vi "DoubleClick.vi"(4 "Point":cluster{"H":T1, "V":T1}, 5 "XRef":refnum<vi>, 6 "State In":T2) -> (0 "Reply":string[](array[string]), 2 "State Out":T2)   [LabVIEW 2015, in "Async-Or-Show.xnode"]
doc: "This ability VI is called when the user double clicks on your XNode. Point is the the location on the XNode that the user clicked relative to the top-left corner of the XNode. A common pattern is to open a configuration dialog when the user double clicks on an XNode, but you may choose to behave differently. Use Reply to inform LabVIEW of any actions it needs to take.\n\nDefault behavior: None.\n\nThis ability provides UI and OS messages are handled."
uses:
  Async-Or-Show.xnode
  State.ctl
  <vilib>/Utility/miscctls.llb/LVRectTypeDef.ctl
  <vilib>/picture/picture.llb/imagedata.ctl
  <vilib>/XNodeSupport/XNodeInt.ctl
  <vilib>/XNodeSupport/NI_XNodeSupport.lvlib
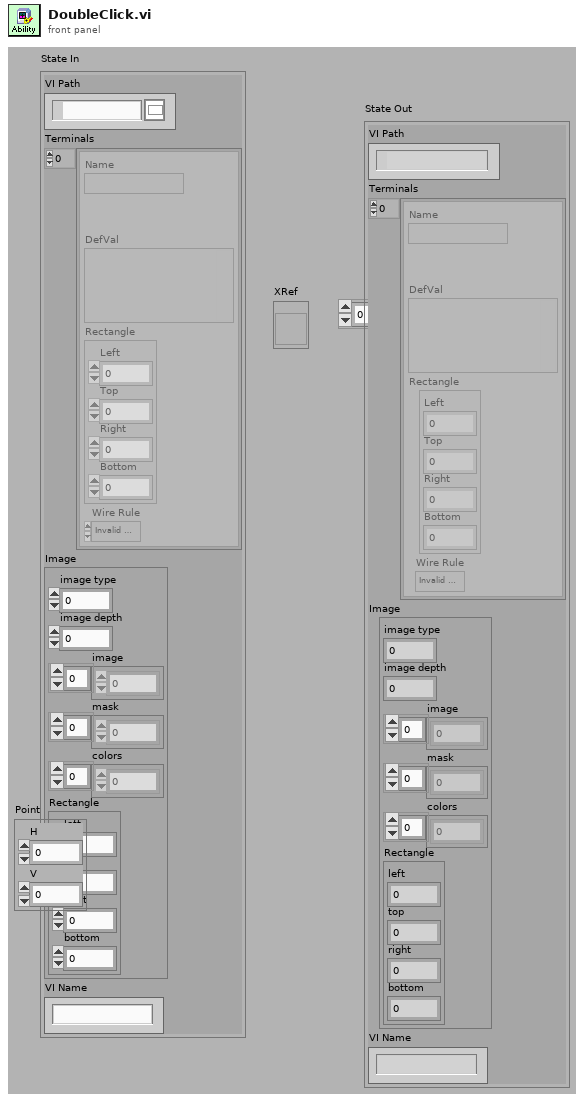
[diagram p1: front panel]
types:
  T1 = typedef "NI_XNodeSupport.lvlib/XNodeInt.ctl" = i32
  T2 = typedef "Async-Or-Show.xnode/State.ctl" = cluster{"VI Path":path, "Terminals":cluster{"Name":string, "DefVal":variant, "Rectangle":T3, "Wire Rule":enum16{"Invalid Wire Rule", "Required", "Recommended", "Optional", "Dynamic Dispatch"}}[], "Image":T4, "VI Name":string}
  T3 = typedef "LVRectTypeDef.ctl" = cluster{"Left":i16, "Top":i16, "Right":i16, "Bottom":i16}
  T4 = typedef "imagedata.ctl" = cluster{"image type":i32, "image depth":i32, "image":u8[], "mask":u8[], "colors":u32[], "Rectangle":cluster{"left":i16, "top":i16, "right":i16, "bottom":i16}}
  T5 = enum16{"Invalid Wire Rule", "Required", "Recommended", "Optional", "Dynamic Dispatch"}[]
  T6 = cluster{"Name":string, "DefVal":variant, "Rectangle":T3, "Wire Rule":enum16{"Invalid Wire Rule", "Required", "Recommended", "Optional", "Dynamic Dispatch"}}[]
  T7 = cluster{"Label.Text":string, "DefVal":variant, "Rectangle":T3, "Wire Rule":enum16{"Invalid Wire Rule", "Required", "Recommended", "Optional", "Dynamic Dispatch"}}[]
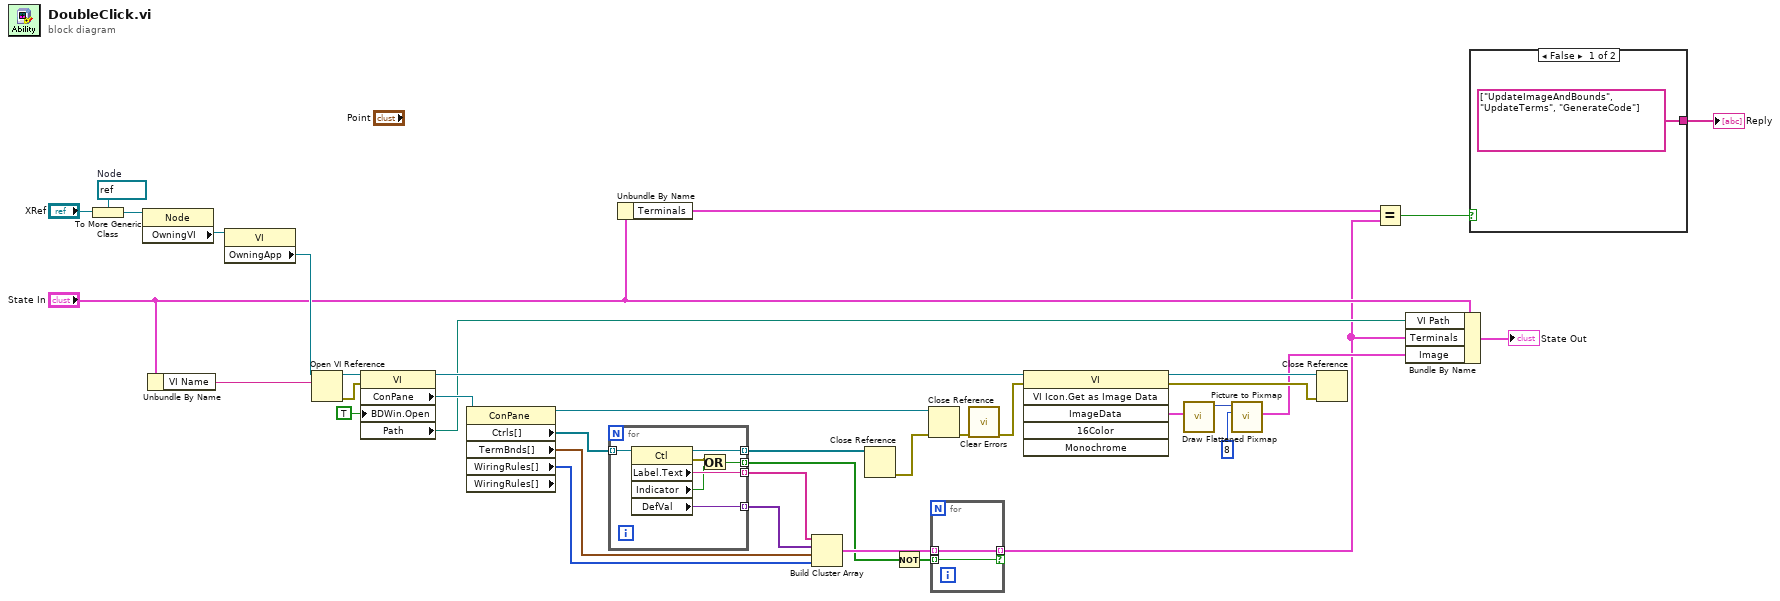
[diagram p0: block diagram]
diagram:
  w31 = refnum<vi> refnum  # Node
  n1 = To More Generic Class(target class=w31, reference="XRef") -> (generic class reference=w30:refnum<vi>)
  n2 = property class="Node"(reference=w30) -> ("OwningVI"=w29:refnum<vi>)  [unwired: 1 in, 2 out]
  n3 = Unbundle By Name("State In") -> ("VI Name"=w34:string)
  n4 = property class="VI"(reference=w29) -> ("OwningApp"=w28:refnum<vi>)  [unwired: 1 in, 2 out]
  n5 = Open VI Reference(application reference (local)=w28, vi path=w34) -> (vi reference=w37:refnum<vi>, error out=w36:errorcluster)  [unwired: 4 in]
  n6 = property class="VI"(reference=w37, error in=w36, "BDWin.Open"=TRUE ("Block Diagram Window:Open")) -> (reference out=w9:refnum<vi>, "ConPane"=w8:refnum<vi>, "Path"=w6:path)  [unwired: 1 out]
  n7 = property class="ConPane" props=["Ctrls[]", "TermBnds[]", "WiringRules[]", "WiringRules[]"](reference=w8) -> (reference out=w16:refnum<vi>, "Ctrls[]"=w27:refnum<vi>[], "TermBnds[]"=w25:T3[], "WiringRules[]"=w26:T5)  [unwired: 1 in, 2 out]
  n8 = for {
    tunnel: w27 -> [w44] mode=indexing
    tunnel: [w43] -> w23 mode=indexing
    tunnel: [w42] -> w24 mode=indexing
    tunnel: [w41] -> w22 mode=indexing
    tunnel: [w38] -> w14 mode=indexing
    n9 = property class="Ctl"(reference=w44) -> (reference out=w41:refnum<vi>, error out=w40:errorcluster, "Label.Text"=w43:string, "Indicator"=w39:bool, "DefVal"=w42:variant)  [unwired: 1 in]
    n10 = Or(x=w40, y=w39) -> (x .or. y?=w38:bool)
  }
  n11 = Unbundle By Name("State In") -> ("Terminals"=w5:T6)
  n12 = Build Cluster Array(w23, w24, w25, w26) -> (w15:T7)
  n13 = Close Reference(reference=w22) -> (error out=w21:errorcluster)  [unwired: 1 in]
  n14 = Not(x=w14) -> (.not. x?=w13:bool[])
  n15 = Close Reference(reference=w16, error in (no error)=w21) -> (error out=w20:errorcluster)
  n16 = for {
    tunnel: w15 -> [w46] mode=indexing
    tunnel: [w46] -> w2 mode=indexing if=w45
    tunnel: w13 -> [w45] mode=indexing
  }
  n17 = call <vilib>:"Clear Errors.vi"("error in (no error)"=w20) -> ("error out"=w17:errorcluster)  [unwired: 5 in, 1 out]
  n18 = invoke class="VI" method="VI Icon.Get as Image Data"(reference=w9, error in=w17) -> (reference out=w19:refnum<vi>, error out=w18:errorcluster, "ImageData"=w12:T4)  [unwired: 4 in, 3 out]
  n19 = call <vilib>:"Draw Flattened Pixmap.vi"("image data"=w12) -> ("new picture"=w11:picture)  [unwired: 8 in]
  n20 = call <vilib>:"Picture to Pixmap.vi"("depth"=8, "picture"=w11) -> ("image data"=w7:T4)  [unwired: 8 in, 1 out]
  n21 = Close Reference(reference=w19, error in (no error)=w18) -> ()  [unwired: 1 out]
  n22 = Equal?(x=w5, y=w2) -> (x = y?=w4:bool)
  n23 = Bundle By Name(cluster="State In", "VI Path"=w6, "Terminals"=w2, "Image"=w7) -> (→"State Out":T2)
  n24 = case shown="False" w4 {
    tunnel: [string[] ["UpdateImageAndBounds", "UpdateTerms", "GenerateCode"] ("Reply") _] -> w1
    frame False {
    }
    frame True {
    }
  }
  "Reply" <- w1
